vi "GenerateList.vi"(8 "error in (no error)":errorcluster, 10 "reference":refnum<vi>, 11 "List in":refnum<class "List.lvclass">) -> (0 "error out":errorcluster, 3 "List out":refnum<class "List.lvclass">)   [LabVIEW 2015, in "List.lvclass"]
uses:
  List.lvclass
  List.lvclass/List.ctl
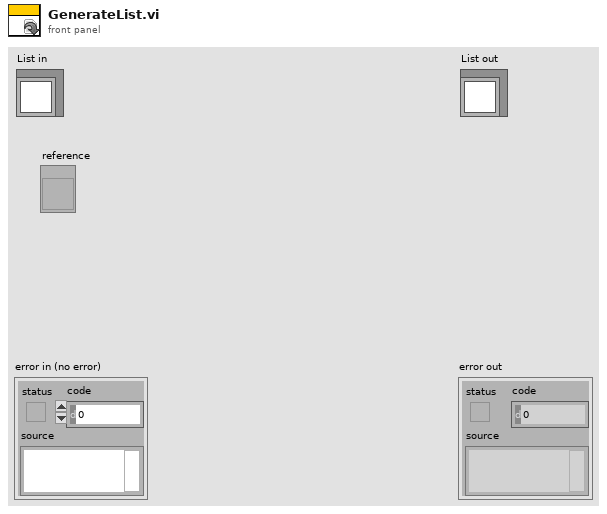
[diagram p1: front panel]
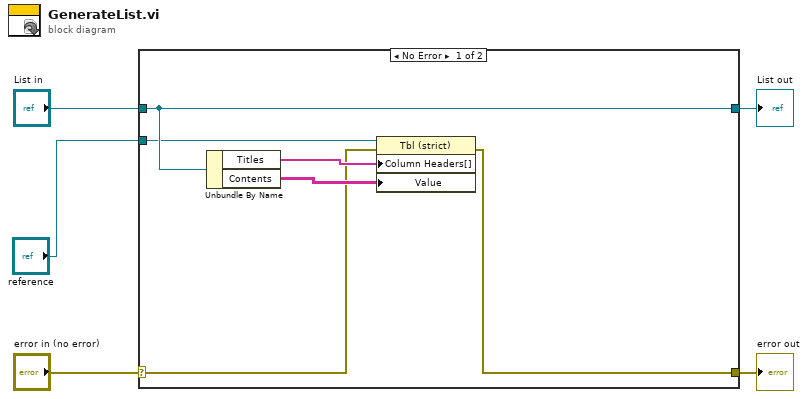
[diagram p0: block diagram]
diagram:
  n1 = case shown="No Error" "error in (no error)" {
    selector: "error in (no error)" -> [w8 w13]
    tunnel: [w7 w13] -> w4
    tunnel: [w11 w12] -> w2
    tunnel: "List in" -> [w11 w12]
    tunnel: "reference" -> [w6 _]
    frame No Error {
      n2 = Unbundle By Name(w11) -> ("Titles"=w10:string[], "Contents"=w9:string[][])
      n3 = property class="Tbl (strict)"(reference=w6, error in=w8, "Column Headers[]"=w10, "Value"=w9) -> (error out=w7:errorcluster)  [unwired: 1 out]
    }
    frame Error {
    }
  }
  "error out" <- w4
  "List out" <- w2
